vi "Write Data ID.vi"(8 "error in":errorcluster, 10 "Data ID":string="GenDataObj", 11 "Data in":refnum<class "Data.lvclass">) -> (0 "error out":errorcluster, 3 "Data out":refnum<class "Data.lvclass">)   [LabVIEW 2014, in "Base Data Class.lvlib" / "Data.lvclass"]
uses:
  Data.lvclass
  Data.lvclass/Data.ctl
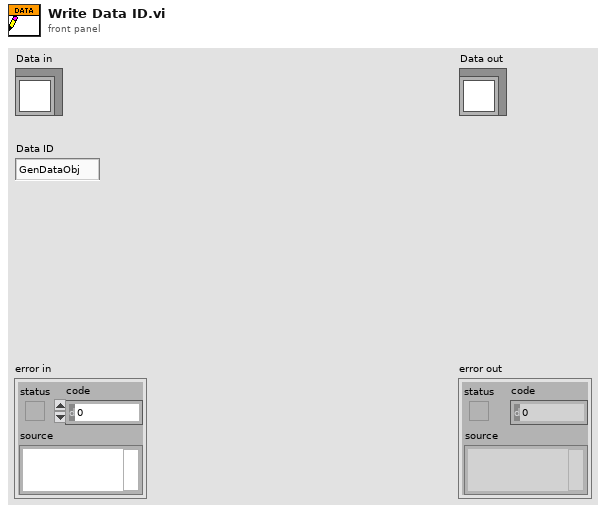
[diagram p1: front panel]
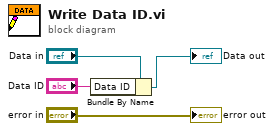
[diagram p0: block diagram]
diagram:
  n1 = Bundle By Name(cluster="Data in", "Data ID"="Data ID") -> (→"Data out":refnum<class "Data.lvclass">)
  "error out" <- "error in"
